vi "GA Set Crd Prm.vi"(8 "error in (no error)":errorcluster caption="错误输入（无错误）", 10 "pCrdPrm":T1, 11 "nCrdNum":i16) -> (0 "error out":errorcluster caption="错误输出", 2 "pCrdPrm out":T1, 3 "function return":i32)   [LabVIEW 2015, in "GAS.lvlib"]
doc: "extern \"C\" __declspec(dllimport) int GA_SetCrdPrm(short nCrdNum,TCrdPrm *pCrdPrm);"
uses:
  <userlib>/BP_GAS/GAS.lvlib
  <userlib>/BP_GAS/GAS.dll
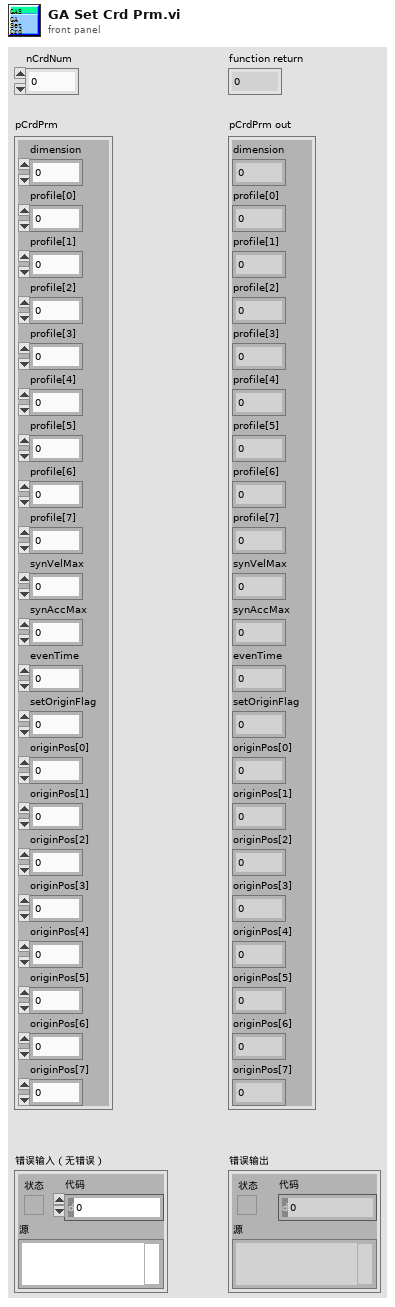
[diagram p1: front panel]
types:
  T1 = cluster{"dimension":i16, "profile[0]":i16, "profile[1]":i16, "profile[2]":i16, "profile[3]":i16, "profile[4]":i16, "profile[5]":i16, "profile[6]":i16, "profile[7]":i16, "synVelMax":dbl, "synAccMax":dbl, "evenTime":i16, "setOriginFlag":i16, "originPos[0]":i32, "originPos[1]":i32, "originPos[2]":i32, "originPos[3]":i32, "originPos[4]":i32, "originPos[5]":i32, "originPos[6]":i32, "originPos[7]":i32}
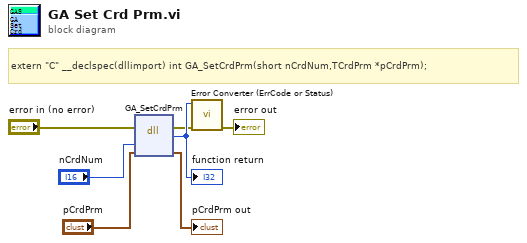
[diagram p0: block diagram]
diagram:
  # "extern \"C\" __declspec(dllimport) int GA_SetCrdPrm(short nCrdNum,TCrdPrm *pCrdPrm);"
  n1 = dll-call lib="E:/Program Files (x86)/National Instruments/LabVIEW 2015/user.lib/BP_GAS/GAS.*" fn="GA_SetCrdPrm"(error in="error in (no error)", "nCrdNum"="nCrdNum", "pCrdPrm"="pCrdPrm") -> (error out=w2:errorcluster, w7:i32, "pCrdPrm"=→"pCrdPrm out":T1)  [unwired: 3 in, 1 out]
  "function return" <- w7
  n2 = call "Error Converter (ErrCode or Status).vi"("error in (no error)"=w2, "error code"=w7) -> ("error out"=→"error out":errorcluster)  [unwired: 9 in]
